vi "Pre Launch Init.vi"(11 "CameraTestingUI in":refnum<class "CameraTestingUI.lvclass">) -> (0 "error out":errorcluster, 3 "CameraTestingUI out":refnum<class "CameraTestingUI.lvclass">)   [LabVIEW 2020, in "CameraTestingUI.lvlib" / "CameraTestingUI.lvclass"]
doc: "(<B>Filename</B>: Actor Framework.lvlib:Actor.lvclass:Pre Launch Init.vi)\n\nDefines behavior that occurs after the Launch Nested Actor method is invoked but before the actor's Actor Core method begins running.\n\nBy default, this method does nothing. A descendant class may override it to define behavior."
uses:
  CameraTestingUI.lvclass
  C:/Program Files (x86)/National Instruments/LabVIEW 2020/vi.lib/ActorFramework/Actor/Actor.lvclass
  Private/TypeDef/PreLaunchInitState.ctl
  CameraTestingUI.lvclass/CameraTestingUI.ctl
  ICameraTesting/TypeDef/Events.ctl
  Camera/ICamera/TypeDef/SnapInfo.ctl
  ICameraTesting/TypeDef/FrameRateValReceived.ctl
  ICameraTesting/TypeDef/ImgTypeValReceived.ctl
  ICameraTesting/TypeDef/ResolutionValReceived.ctl
  ICameraTesting/TypeDef/VideoOptCodesUpdated.ctl
  ICameraTesting/TypeDef/VideoOptionsInfo.ctl
  ICameraTesting/TypeDef/StatusUpdated.ctl
  ICameraTesting/TypeDef/StatusRecord.ctl
  ICameraTesting/TypeDef/VideoBufferUpdate.ctl
  Private/TypeDef/VideoLoopCamTestEvn.ctl
  Private/TypeDef/HelperLoopCamTestEvn.ctl
  <vilib>/ActorFramework/Actor/Actor.lvclass/Actor.ctl
  <vilib>/ActorFramework/Message Enqueuer/Message Priority.ctl
  <vilib>/ActorFramework/Message Enqueuer/Message Enqueuer.lvclass/Message Enqueuer.ctl
  <vilib>/ActorFramework/Message Enqueuer/Enqueue.vi
  <vilib>/ActorFramework/Message Enqueuer/Init from Existing Queue.vi
  ICameraTesting/ICameraTesting Messages/GetEvents Msg/GetEvents Msg.lvclass
  C:/Program Files (x86)/National Instruments/LabVIEW 2020/vi.lib/ActorFramework/Message/Message.lvclass
  CameraTestingUI Messages/Init Msg/Init Msg.lvclass
  <vilib>/ActorFramework/Message Priority Queue/Priority Enqueue.vi
  <vilib>/ActorFramework/Message Enqueuer/Message Enqueuer.lvclass
  <vilib>/ActorFramework/Actor/Actor.lvclass
  Camera/ICamera/TypeDef/ICamera_typedef.lvlib
  ICameraTesting/TypeDef/ICameraTesting_typedef.lvlib
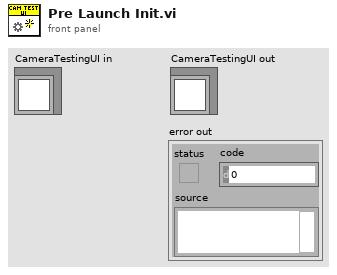
[diagram p1: front panel]
types:
  T1 = typedef "CameraTestingUI.lvlib/CameraTestingUI.lvclass/PreLaunchInitState.ctl" = enum16{"Create Events", "Registration Events", "Get Controller Events", "Call Internal Init"}
  T2 = typedef "Actor Framework.lvlib/Message Enqueuer.lvclass/Message Priority.ctl" = enum16{"Low", "Normal", "High"}
  T3 = typedef "ICameraTesting_typedef.lvlib/Events.ctl" = cluster{"NewSnapData":refnum<user-event>, "FrameRateValReceived":T4, "ImgTypeValReceived":T5, "ResolutionValReceived":T6, "VideoOptInfoUpdated":T7, "StatusUpdated":T8, "VideoBufferUpdate":T9}
  T4 = typedef "ICameraTesting_typedef.lvlib/FrameRateValReceived.ctl" = refnum<user-event>
  T5 = typedef "ICameraTesting_typedef.lvlib/ImgTypeValReceived.ctl" = refnum<user-event>
  T6 = typedef "ICameraTesting_typedef.lvlib/ResolutionValReceived.ctl" = refnum<user-event>
  T7 = typedef "ICameraTesting_typedef.lvlib/VideoOptCodesUpdated.ctl" = refnum<user-event>
  T8 = typedef "ICameraTesting_typedef.lvlib/StatusUpdated.ctl" = refnum<user-event>
  T9 = typedef "ICameraTesting_typedef.lvlib/VideoBufferUpdate.ctl" = refnum<user-event>
  T10 = typedef "CameraTestingUI.lvlib/CameraTestingUI.lvclass/VideoLoopCamTestEvn.ctl" = cluster{"VideoBufferUpdate":T9}
  T11 = typedef "CameraTestingUI.lvlib/CameraTestingUI.lvclass/HelperLoopCamTestEvn.ctl" = cluster{"NewSnapData":refnum<user-event>, "FrameRateValReceived":T4, "ImgTypeValReceived":T5, "ResolutionValReceived":T6, "VideoOptInfoUpdated":T7, "StatusUpdated":T8}
  T12 = typedef "CameraTestingUI.lvlib/CameraTestingUI.lvclass/PrivateEvents.ctl" = cluster{"UpdCamTestEvntRegRef":T13, "QuitActorEnv":T14}
  T13 = typedef "CameraTestingUI.lvlib/CameraTestingUI.lvclass/UpdCamTestEvntRegRef.ctl" = refnum<user-event>
  T14 = typedef "CameraTestingUI.lvlib/CameraTestingUI.lvclass/QuitActorEvn.ctl" = refnum<user-event>
  T15 = typedef "CameraTestingUI.lvlib/CameraTestingUI.lvclass/HelperLoopEvntRegRef.ctl" = refnum<event-registration>
  T16 = typedef "CameraTestingUI.lvlib/CameraTestingUI.lvclass/VideoLoopEnvRgstRef.ctl" = refnum<event-registration>
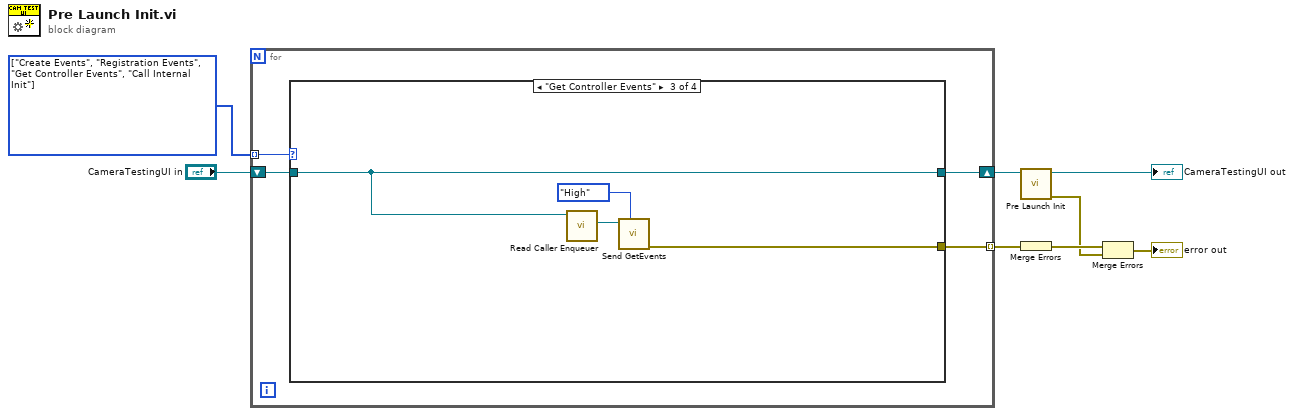
[diagram p0: block diagram]
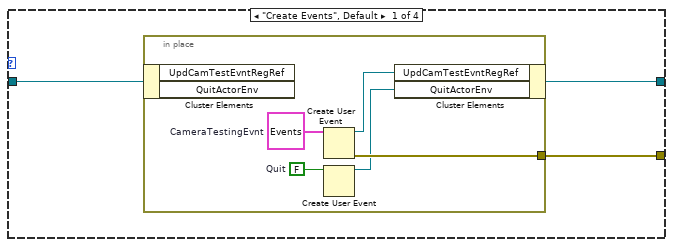
[diagram p2: hidden frame]
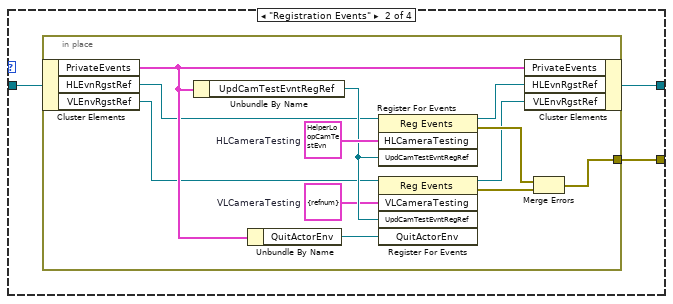
[diagram p3: hidden frame]
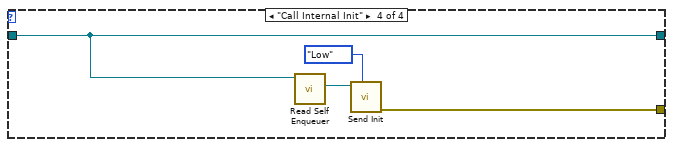
[diagram p4: hidden frame]
diagram:
  w7 = T1[] [enum."Create Events", enum."Registration Events", enum."Get Controller Events", enum."Call Internal Init"] items=["Create Events", "Registration Events", "Get Controller Events", "Call Internal Init"]
  n1 = for {
    tunnel: [w10] -> w1 mode=indexing
    shift-right: [w11] -> w6
    shift-left: "CameraTestingUI in" -> [w12]
    tunnel: w7 -> [w9] mode=indexing
    n2 = case shown="\"Get Controller Events\"" w9 {
      tunnel: w12 -> [w15 w23 w39 w43]
      tunnel: [w14 w22 w39 w43] -> w11
      tunnel: [w13 w21 w38 w42] -> w10
      frame "Create Events", Default {
        n3 = in-place {
          in-place-border: [w18] -> w13
          w17 = FALSE  # Quit
          w20 = T3 {"NewSnapData"=refnum, "FrameRateValReceived"=refnum, "ImgTypeValReceived"=refnum, "ResolutionValReceived"=refnum, "VideoOptInfoUpdated"=refnum, "StatusUpdated"=refnum, "VideoBufferUpdate"=refnum}  # CameraTestingEvnt
          n4 = in-place-cluster #1(w15) -> ()  [unwired: 2 out]
          n5 = Create User Event(user event datatype=w20) -> (user event=w19:refnum<user-event>, error out=w18:errorcluster)  [unwired: 1 in]
          n6 = Create User Event(user event datatype=w17) -> (user event=w16:refnum<user-event>)  [unwired: 1 in, 1 out]
          n7 = in-place-cluster #1("UpdCamTestEvntRegRef"=w19, "QuitActorEnv"=w16) -> (w14:refnum<class "CameraTestingUI.lvclass">)
        }
      }
      frame "Registration Events" {
        n8 = in-place {
          in-place-border: [w34] -> w21
          w31 = T10 {"VideoBufferUpdate"=refnum}  # VLCameraTesting
          w33 = T11 {"NewSnapData"=refnum, "FrameRateValReceived"=refnum, "ImgTypeValReceived"=refnum, "ResolutionValReceived"=refnum, "VideoOptInfoUpdated"=refnum, "StatusUpdated"=refnum}  # HLCameraTesting
          n9 = in-place-cluster #2(w23) -> ("PrivateEvents"=w29:T12, "HLEvnRgstRef"=w25:T15, "VLEnvRgstRef"=w27:T16)
          n10 = Unbundle By Name(w29) -> ("UpdCamTestEvntRegRef"=w32:T13)
          n11 = Unbundle By Name(w29) -> ("QuitActorEnv"=w28:T14)
          n12 = register-events(reference=w25, w33, w32) -> (reference out=w24:T15, error out=w35:errorcluster)  [unwired: 1 in]
          n13 = register-events(reference=w27, w31, w32, w28) -> (reference out=w26:T16, error out=w30:errorcluster)  [unwired: 1 in]
          n14 = in-place-cluster #2("PrivateEvents"=w29, "HLEvnRgstRef"=w24, "VLEnvRgstRef"=w26) -> (w22:refnum<class "CameraTestingUI.lvclass">)
          n15 = Merge Errors(w35, w30) -> (w34:errorcluster)
        }
      }
      frame "Get Controller Events" {
        n16 = call <vilib>:"Read Caller Enqueuer.vi"("Actor"=w39) -> ("Caller Enqueuer"=w37:refnum<class "Message Enqueuer.lvclass">)  [unwired: 10 in]
        n17 = call "Send GetEvents.vi"("Message Priority (Normal)"=Message_Priority."High", "Message Enqueuer"=w37) -> ("error out"=w38:errorcluster)  [unwired: 8 in, 1 out]
      }
      frame "Call Internal Init" {
        n18 = call <vilib>:"Read Self Enqueuer.vi"("Actor"=w43) -> ("Self Enqueuer"=w41:refnum<class "Message Enqueuer.lvclass">)  [unwired: 10 in]
        n19 = call "Send Init.vi"("Message Priority (Normal)"=Message_Priority."Low", "Message Enqueuer"=w41) -> ("error out"=w42:errorcluster)  [unwired: 8 in, 1 out]
      }
    }
  }
  n20 = call-parent "Pre Launch Init.vi"("Actor in"=w6) -> ("error out"=w3:errorcluster, "Actor out"=→"CameraTestingUI out":refnum<class "CameraTestingUI.lvclass">)  [unwired: 9 in]
  n21 = Merge Errors(w1) -> (w4:errorcluster)
  n22 = Merge Errors(w4, w3) -> (→"error out":errorcluster)
